vi "RPC Method TemperatureControllerService_Configure.vi"(8 "error in (no error)":errorcluster, 10 "Request Data":T2, 11 "gRPC Client in":refnum<class "TempController_client.lvclass">) -> (0 "error out":errorcluster, 2 "Response Data":T1, 3 "gRPC Client out":refnum<class "TempController_client.lvclass">)   [LabVIEW 2019, in "TempController_client.lvlib" / "TempController_client.lvclass"]
uses:
  TempController_client.lvclass
  RPC Messages/ControllerSettingsRequest/ControllerSettingsRequest_Data.ctl
  RPC Messages/EmptyResponse/EmptyResponse_Data.ctl
  TempController_client.lvclass/TempController_client.ctl
  fa22ca14-33b2-4bc3-8699-3f27c9b27c9c.vi
  <vilib>/gRPC/LabVIEW gRPC Library/Server API/Server/Get Server DLL Path.vi
panel:
  out "return type":i32
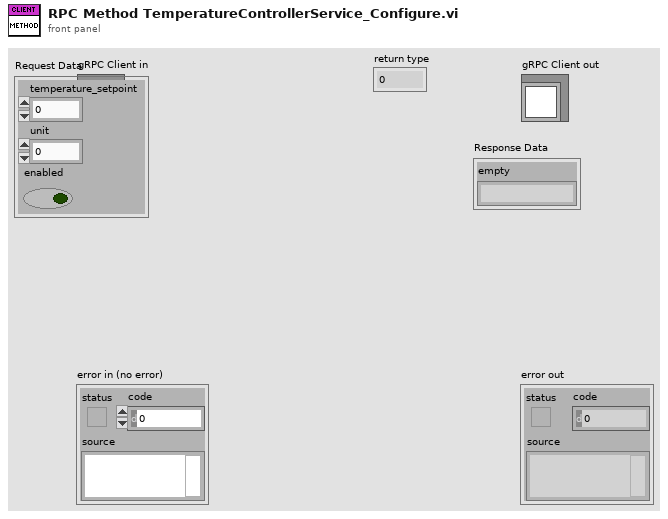
[diagram p1: front panel]
types:
  T1 = typedef "TempController_client.lvlib/TempController_client.lvclass/EmptyResponse_Data.ctl" = cluster{"empty":string}
  T2 = typedef "TempController_client.lvlib/TempController_client.lvclass/ControllerSettingsRequest_Data.ctl" = cluster{"temperature_setpoint":dbl, "unit":i32, "enabled":bool}
  T3 = typedef "gprc-lvsupport-release.lvlib/grpcId.ctl" = u64
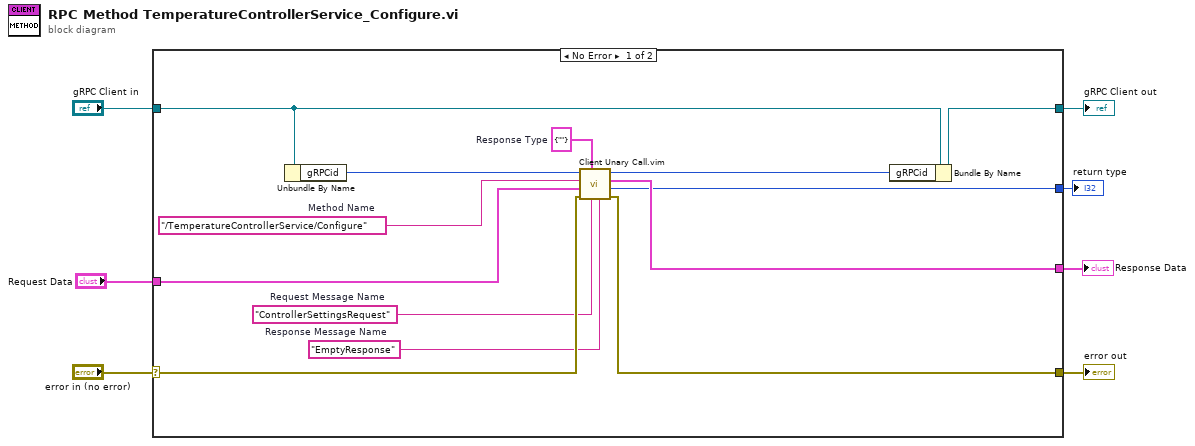
[diagram p0: block diagram]
diagram:
  n1 = case shown="No Error" "error in (no error)" {
    selector: "error in (no error)" -> [w16 w22]
    tunnel: [w15 w22] -> w6
    tunnel: [w17 w21] -> w4
    tunnel: "gRPC Client in" -> [w19 w21]
    tunnel: "Request Data" -> [w13 _]
    tunnel: [w12 _] -> w2
    tunnel: [w8 _] -> w1
    frame No Error {
      w9 = "EmptyResponse"  # Response Message Name
      w10 = "ControllerSettingsRequest"  # Request Message Name
      w11 = T1 {"empty"=""}  # Response Type
      w14 = "/TemperatureControllerService/Configure"  # Method Name
      n2 = Unbundle By Name(w19) -> ("gRPCid"=w20:T3)
      n3 = call "Client Unary Call.vim"("Response Message Name"=w9, "Request Message Name"=w10, "Response Type"=w11, "error in (no error)"=w16, "Request Data"=w13, "Method Name"=w14, "Client Ref"=w20) -> ("error out"=w15:errorcluster, "return type"=w8:i32, "Response Data"=w12:T1, "Client Ref Out"=w18:u64)  [unwired: 1 in]
      n4 = Bundle By Name(cluster=w19, "gRPCid"=w18) -> (w17:refnum<class "TempController_client.lvclass">)
    }
    frame Error {
    }
  }
  "error out" <- w6
  "gRPC Client out" <- w4
  "Response Data" <- w2
  "return type" <- w1
